vi "Read Lockout.vi"(0 "VISA resource name":refnum<visa-resource-name>, 3 "Password (pppp)":i32 format="%04.0f", 7 "error in (no error)":errorcluster) -> (14 "Dispense Vacuum?":bool, 16 "Memory Cell Selection?":bool, 17 "Auto Increment Reset?":bool, 18 "Dispense Time?":bool, 19 "Alarms Reset?":bool, 20 "VISA resource name out":refnum<visa-resource-name>, 21 "Dispense Mode Change?":bool, 22 "Dispense Pressure?":bool, 23 "Deposit Counter Selection?":bool, 24 "AI Mode Selection?":bool, 25 "Main Menu Selection?":bool, 26 "Alarm Options Menu Selection?":bool, 27 "error out":errorcluster)   [LabVIEW 2016, in "EFD Ultimus V.lvlib"]
doc: "Reads the operator lockout settings from the Ultimus V. 'D0' is the number zero (0).\n\nHost Format: EH--PApppp\npppp: Four digit password. This needs to match the password set on the dispenser. The dispenser will return an error if incorrect.\n\nReturn Format: D0DTtDPpDVvMmDCcDMdAIaARuALbMMePUfVUgLAhCLjCOkAMn\n\nt: lock out dispense time: '1'=lockout, '0'=enabled\np: lockout dispense pressure: \nv: lockout dispense vacuum: \nm: lockout memory cell selection: \nc: lockout deposit counter selection:\nd: lockout dispense mode change: \na: lockout Auto Increment Mode selection: \nu: lockout Auto Increment Reset:\nb: lockout Alarms Reset:\ne: lockout Main Menu selection: \nf: lockout Pressure Unit Menu selection: \ng: lockout Vacuum Unit Menu selection: \nh: lockout Language Menu selection: \nj: lockout Set Clock/Date Menu selection: \nk: lockout Set Communications Menu selection: \nn: lockout Alarm Options Menu selection:"
uses:
  EFD Ultimus V.lvlib
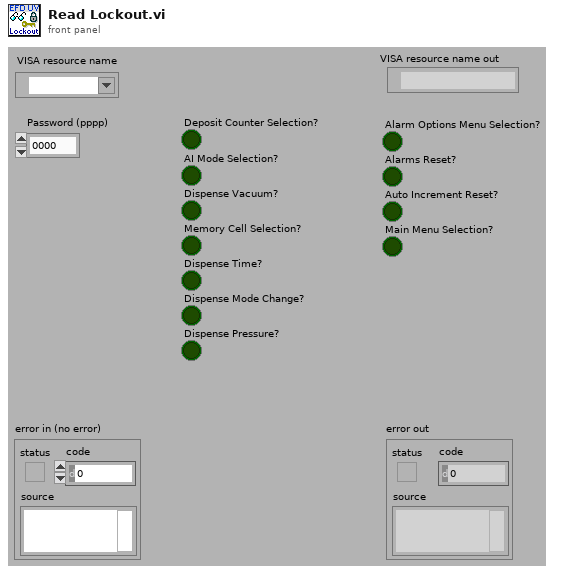
[diagram p1: front panel]
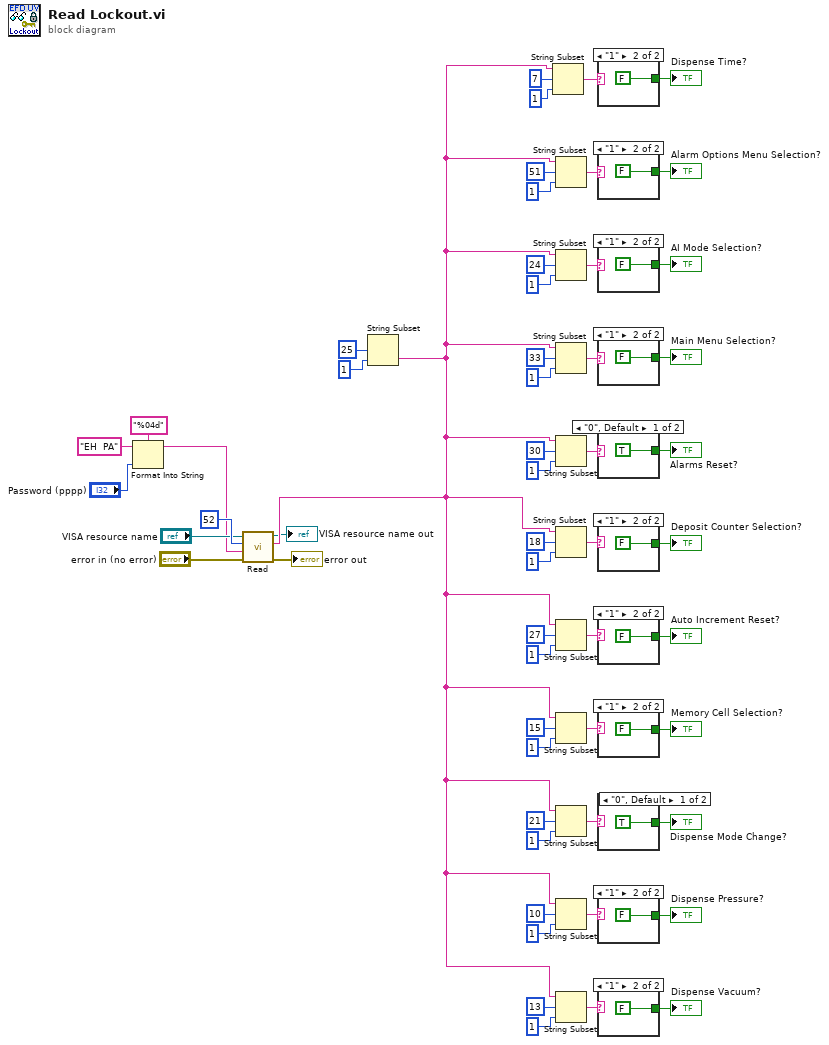
[diagram p0: block diagram]
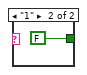
[diagram p2: hidden frame]
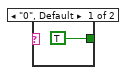
[diagram p3: hidden frame]
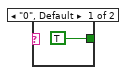
[diagram p4: hidden frame]
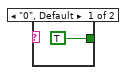
[diagram p5: hidden frame]
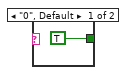
[diagram p6: hidden frame]
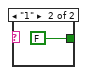
[diagram p7: hidden frame]
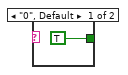
[diagram p8: hidden frame]
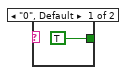
[diagram p9: hidden frame]
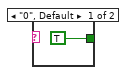
[diagram p10: hidden frame]
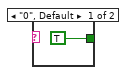
[diagram p11: hidden frame]
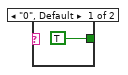
[diagram p12: hidden frame]
diagram:
  n1 = Format Into String(format string="%04d", initial string="EH  PA" ("Command To Write"), "Password (pppp)") -> (resulting string=w3:string)  [unwired: 1 in, 1 out]
  n2 = call "Read.vi"("error in (no error)"="error in (no error)", "Command To Write"=w3, "Bytes to Read (11)"=u32 52 ("Bytes to Read from Buffer"), "VISA resource name"="VISA resource name") -> ("error out"=→"error out":errorcluster, "Ultimus V Feedback Data"=w11:string, "VISA resource name out"=→"VISA resource name out":refnum<visa-resource-name>)  [unwired: 5 out]
  n3 = String Subset(string=w11, offset (0)=25, length (rest)=1 ("length (rest)")) -> ()  [unwired: 1 out]
  n4 = String Subset(string=w11, offset (0)=7, length (rest)=1 ("length (rest)")) -> (substring=w35:string)
  n5 = String Subset(string=w11, offset (0)=51, length (rest)=1 ("length (rest)")) -> (substring=w43:string)
  n6 = String Subset(string=w11, offset (0)=24, length (rest)=1 ("length (rest)")) -> (substring=w40:string)
  n7 = String Subset(string=w11, offset (0)=33, length (rest)=1 ("length (rest)")) -> (substring=w42:string)
  n8 = String Subset(string=w11, offset (0)=30, length (rest)=1 ("length (rest)")) -> (substring=w1:string)
  n9 = String Subset(string=w11, offset (0)=18, length (rest)=1 ("length (rest)")) -> (substring=w38:string)
  n10 = String Subset(string=w11, offset (0)=27, length (rest)=1 ("length (rest)")) -> (substring=w41:string)
  n11 = String Subset(string=w11, offset (0)=15 ("length (rest)"), length (rest)=1 ("length (rest)")) -> (substring=w37:string)
  n12 = String Subset(string=w11, offset (0)=21, length (rest)=1 ("length (rest)")) -> (substring=w39:string)
  n13 = String Subset(string=w11, offset (0)=10, length (rest)=1 ("length (rest)")) -> (substring=w44:string)
  n14 = String Subset(string=w11, offset (0)=13, length (rest)=1 ("length (rest)")) -> (substring=w36:string)
  n15 = case shown="\"1\"" w35 {
    tunnel: [TRUE FALSE] -> w50
    frame "0", Default {
    }
    frame "1" {
    }
  }
  "Dispense Time?" <- w50
  n16 = case shown="\"1\"" w43 {
    tunnel: [TRUE FALSE] -> w47
    frame "0", Default {
    }
    frame "1" {
    }
  }
  "Alarm Options Menu Selection?" <- w47
  n17 = case shown="\"1\"" w40 {
    tunnel: [TRUE FALSE] -> w55
    frame "0", Default {
    }
    frame "1" {
    }
  }
  "AI Mode Selection?" <- w55
  n18 = case shown="\"1\"" w42 {
    tunnel: [TRUE FALSE] -> w46
    frame "0", Default {
    }
    frame "1" {
    }
  }
  "Main Menu Selection?" <- w46
  n19 = case shown="\"0\", Default" w1 {
    tunnel: [TRUE FALSE] -> w54
    frame "0", Default {
    }
    frame "1" {
    }
  }
  "Alarms Reset?" <- w54
  n20 = case shown="\"1\"" w38 {
    tunnel: [TRUE FALSE] -> w49
    frame "0", Default {
    }
    frame "1" {
    }
  }
  "Deposit Counter Selection?" <- w49
  n21 = case shown="\"1\"" w41 {
    tunnel: [TRUE FALSE] -> w48
    frame "0", Default {
    }
    frame "1" {
    }
  }
  "Auto Increment Reset?" <- w48
  n22 = case shown="\"1\"" w37 {
    tunnel: [TRUE FALSE] -> w52
    frame "0", Default {
    }
    frame "1" {
    }
  }
  "Memory Cell Selection?" <- w52
  n23 = case shown="\"0\", Default" w39 {
    tunnel: [TRUE FALSE] -> w53
    frame "0", Default {
    }
    frame "1" {
    }
  }
  "Dispense Mode Change?" <- w53
  n24 = case shown="\"1\"" w44 {
    tunnel: [TRUE FALSE] -> w51
    frame "0", Default {
    }
    frame "1" {
    }
  }
  "Dispense Pressure?" <- w51
  n25 = case shown="\"1\"" w36 {
    tunnel: [TRUE FALSE] -> w56
    frame "0", Default {
    }
    frame "1" {
    }
  }
  "Dispense Vacuum?" <- w56
